vi "Timestamp to Unix epoch time.vi"(10 "Precision (ns)":T1=enum."Nanoseconds", 11 "Timestamp":timestamp format="%<%H:%M:%S%3u\n%Y/%m/%d>T") -> (3 "Unix epoch time":u64)   [LabVIEW 2018, in "InfluxDB Client.lvlib"]
doc: "Convert the LabVIEW timestamp format to Unix epoch time."
uses:
  Controls/Precision.ctl
  InfluxDB Client.lvlib
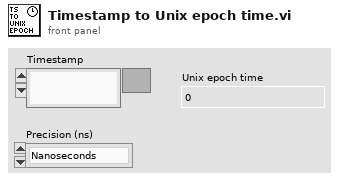
[diagram p1: front panel]
types:
  T1 = typedef "InfluxDB Client.lvlib/Precision.ctl" = enum16{"Seconds", "Milliseconds", "Nanoseconds"}
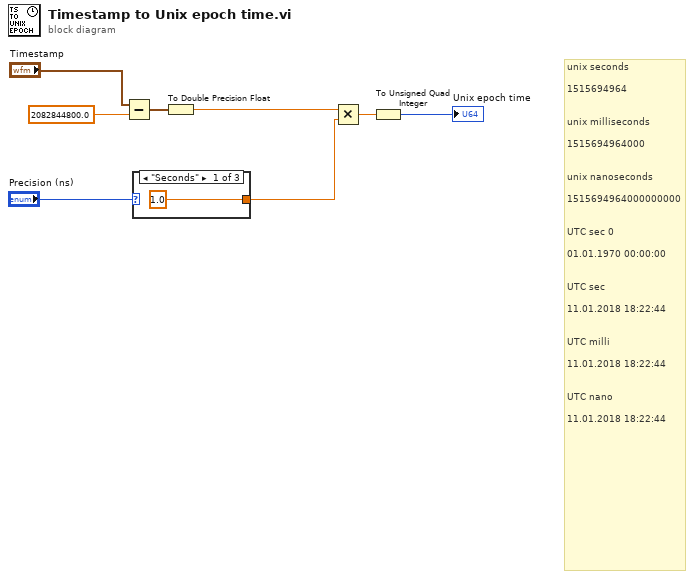
[diagram p0: block diagram]
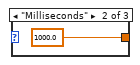
[diagram p2: hidden frame]
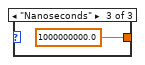
[diagram p3: hidden frame]
diagram:
  # "unix seconds\n\n1515694964 \n\n\nunix milliseconds\n\n1515694964000 \n\n\nunix nanoseconds\n\n1515694964000000000 \n\n\nUTC sec 0\n\n01.01.1970 00:00:00 \n\n\nUTC sec\n\n11.01.2018 18:22:44 \n\n\nUTC milli\n\n11.01.2018 18:22:44 \n\n\nUTC nano\n\n11.01.2018 18:22:44"
  n1 = Subtract(x="Timestamp", y=2082844800.0) -> (x-y=w5:timestamp)
  n2 = case shown="\"Seconds\"" "Precision (ns)" {
    tunnel: [1.0 ("Database name") 1000.0 ("Database name") 1000000000.0 ("Database name")] -> w2
    frame "Seconds" {
    }
    frame "Milliseconds" {
    }
    frame "Nanoseconds" {
    }
  }
  n3 = To Double Precision Float(number=w5) -> (double precision float=w7:dbl)
  n4 = Multiply(x=w7, y=w2) -> (x*y=w6:dbl)
  n5 = To Unsigned Quad Integer(1:w6) -> (0:→"Unix epoch time":u64)
